vi "example_2.vi"() -> ()   [LabVIEW 2021]
uses:
  <vilib>/Analysis/baseanly.llb/Mean (DBL).vi
  <vilib>/Analysis/NI_AALBase.lvlib
panel:
  out "Time with dll":u32
  out "Time with \"On\"":u32
  out "Time with \"Auto\"":u32
  in  "Time dimensions":bool
  out "MAE Theil-Sen (Off)":dbl format="%0.2f"
  out "MAE Theil-Sen (Auto)":dbl format="%0.2f"
  out "XY Graph":cluster{dbl[], dbl[]}[](graph)
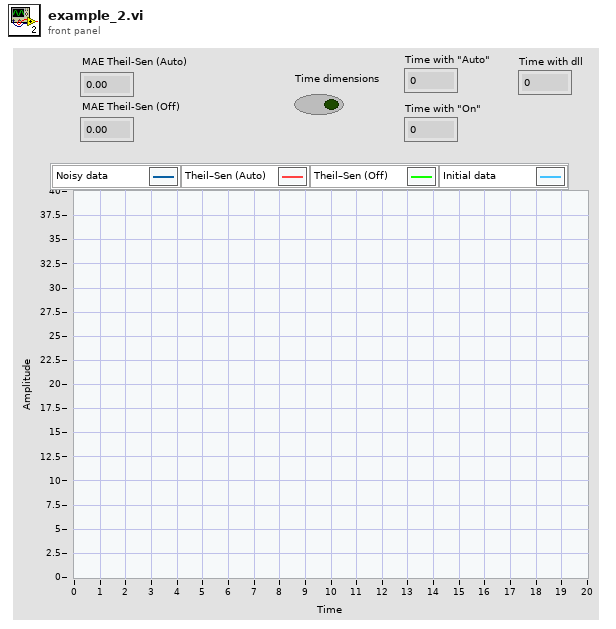
[diagram p1: front panel]
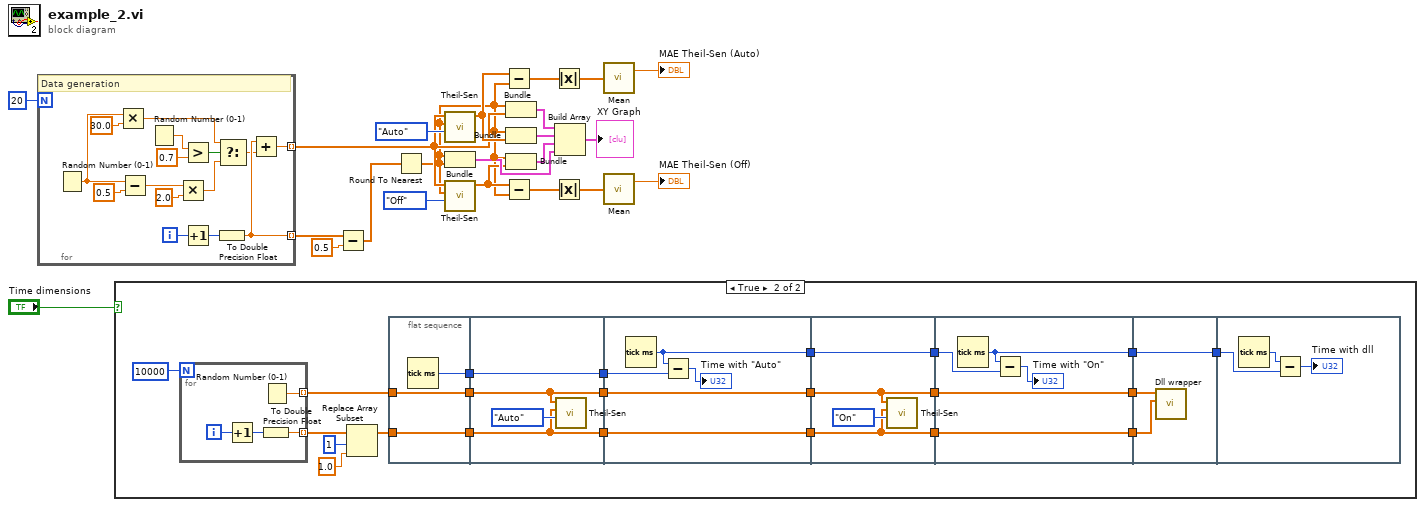
[diagram p0: block diagram]
diagram:
  n1 = for {
    N: 20 -> [_]
    tunnel: [w25] -> w15 mode=indexing
    tunnel: [w23] -> w2 mode=indexing
    i -> [w35]
    # "Data generation"
    n2 = Random Number (0-1)() -> (number: 0 to 1=w27:dbl)
    n3 = Multiply(x=w27, y=30.0 ("t")) -> (x*y=w26:dbl)
    n4 = Subtract(x=w27, y=0.5) -> (x-y=w37:dbl)
    n5 = Random Number (0-1)() -> (number: 0 to 1=w33:dbl)
    n6 = Multiply(x=w37, y=2.0) -> (x*y=w30:dbl)
    n7 = Greater?(x=w33, y=0.7) -> (0:w29:bool)
    n8 = Increment(x=w35) -> (x+1=w34:i32)
    n9 = To Double Precision Float(number=w34) -> (double precision float=w25:dbl)
    n10 = Select(t=w26, s=w29, f=w30) -> (s? t:f=w24:dbl)
    n11 = Add(x=w25, y=w24) -> (x+y=w23:dbl)
  }
  n12 = case shown="True" "Time dimensions" {
    frame False {
    }
    frame True {
      n13 = for {
        N: 10000 -> [_]
        tunnel: [w61] -> w57 mode=indexing
        tunnel: [w60] -> w47 mode=indexing
        i -> [w62]
        n14 = Increment(x=w62) -> (x+1=w63:i32)
        n15 = To Double Precision Float(number=w63) -> (double precision float=w60:dbl)
        n16 = Random Number (0-1)() -> (number: 0 to 1=w61:dbl)
      }
      n17 = Replace Array Subset(array=w47, new element=1.0 ("new element/subarray"), index=1) -> (w44:dbl[])
      n18 = flat-sequence {
        tunnel: [w66] -> w58
        tunnel: w57 -> [w66]
        tunnel: w44 -> [w65]
        tunnel: [w65] -> w56
        tunnel: [w64] -> w51
        tunnel: w58 -> [w67]
        tunnel: w56 -> [w68]
        tunnel: [w68] -> w54
        tunnel: [w67] -> w53
        tunnel: w51 -> [w69]
        tunnel: [w69] -> w50
        tunnel: [w75] -> w55
        tunnel: w54 -> [w75]
        tunnel: w53 -> [w74]
        tunnel: [w74] -> w52
        tunnel: w50 -> [w73]
        tunnel: [w71] -> w49
        tunnel: w55 -> [w76]
        tunnel: w52 -> [w77]
        tunnel: w49 -> [w78]
        tunnel: [w78] -> w48
        tunnel: [w77] -> w43
        tunnel: [w76] -> w41
        tunnel: w48 -> [w84]
        tunnel: w43 -> [w82]
        tunnel: [w82] -> w42
        tunnel: w41 -> [w81]
        tunnel: [w81] -> w40
        tunnel: [w80] -> w39
        tunnel: w42 -> [w87]
        tunnel: w40 -> [w86]
        tunnel: w39 -> [w85]
        tunnel: [w85] -> w38
        tunnel: w38 -> [w89]
        frame #0 {
          n19 = Tick Count (ms)() -> (millisecond timer value=w64:u32)
        }
        frame #1 {
          n20 = call "Theil-Sen.vi"("Sen parameter (Auto)"=enum16{"Auto", "On", "Off"}."Auto" ("Sen parameter"), "input_X"=w68, "input_Y"=w67) -> ()  [unwired: 3 in, 4 out]
        }
        frame #2 {
          n21 = Tick Count (ms)() -> (millisecond timer value=w71:u32)
          n22 = Subtract(x=w71, y=w73) -> (x-y=→"Time with \"Auto\"":u32)
        }
        frame #3 {
          n23 = call "Theil-Sen.vi"("Sen parameter (Auto)"=enum16{"Auto", "On", "Off"}."On" ("Sen parameter"), "input_X"=w76, "input_Y"=w77) -> ()  [unwired: 3 in, 4 out]
        }
        frame #4 {
          n24 = Tick Count (ms)() -> (millisecond timer value=w80:u32)
          n25 = Subtract(x=w80, y=w84) -> (x-y=→"Time with \"On\"":u32)
        }
        frame #5 {
          n26 = call "Dll wrapper.vi"("X"=w86, "Y"=w87) -> ()  [unwired: 5 in, 5 out]
        }
        frame #6 {
          n27 = Tick Count (ms)() -> (millisecond timer value=w90:u32)
          n28 = Subtract(x=w90, y=w89) -> (x-y=→"Time with dll":u32)
        }
      }
    }
  }
  n29 = Subtract(x=w15, y=0.5) -> (x-y=w13:dbl[])
  n30 = Round To Nearest(number=w13) -> (nearest integer value=w1:dbl[])
  n31 = call "Theil-Sen.vi"("Sen parameter (Auto)"=enum16{"Auto", "On", "Off"}."Auto" ("Sen parameter"), "input_X"=w1, "input_Y"=w2) -> ("output_Y"=w11:dbl[])  [unwired: 3 in, 3 out]
  n32 = Bundle(w1, w1) -> (w19:cluster{dbl[], dbl[]})  [unwired: 1 in]
  n33 = call "Theil-Sen.vi"("Sen parameter (Auto)"=enum16{"Auto", "On", "Off"}."Off" ("Sen parameter"), "input_X"=w1, "input_Y"=w2) -> ("output_Y"=w4:dbl[])  [unwired: 3 in, 3 out]
  n34 = Subtract(x=w11, y=w1) -> (x-y=w10:dbl[])
  n35 = Subtract(x=w4, y=w1) -> (x-y=w5:dbl[])
  n36 = Bundle(w1, w2) -> (w22:cluster{dbl[], dbl[]})  [unwired: 1 in]
  n37 = Bundle(w1, "output_Y"=w11) -> (w21:cluster{dbl[], "output_Y":dbl[]})  [unwired: 1 in]
  n38 = Bundle(w1, "output_Y"=w4) -> (w16:cluster{dbl[], "output_Y":dbl[]})  [unwired: 1 in]
  n39 = Absolute Value(x=w10) -> (abs(x)=w9:dbl[])
  n40 = Absolute Value(x=w5) -> (abs(x)=w6:dbl[])
  n41 = Build Array(w22, w21, w16, w19) -> (→"XY Graph":cluster{dbl[], "output_Y":dbl[]}[])
  n42 = call-poly <vilib>:"Mean.vi"("X"=w9) -> ("mean"=→"MAE Theil-Sen (Auto)":dbl)  [unwired: 1 out]
  n43 = call-poly <vilib>:"Mean.vi"("X"=w6) -> ("mean"=→"MAE Theil-Sen (Off)":dbl)  [unwired: 1 out]
